vi "Get Cursor Info.vi"(8 "error in (no error)":errorcluster) -> (0 "error out":errorcluster, 1 "Image":T1, 2 "Hot Spot":cluster{"x":i32, "y":i32}, 3 "Position":cluster{"x":i32, "y":i32}, 4 "Drawn Image":picture)   [LabVIEW 2020, in "MacroAssert.lvlib" / "Win Util.lvlib"]
doc: "Originally found here.\n\nhttps://decibel.ni.com/content/docs/DOC-15261\n\nModified to get the image in a different way using the save to buffer, along with PNG conversion. Also got the position from the DLL call, and clear error if the data returned looks good.\n\n-----\nBrian Hoover (hooovahh)"
uses:
  Win Util.lvlib
  <vilib>/picture/picture.llb/imagedata.ctl
  System.Windows.Forms
  System.Drawing
  user32.dll
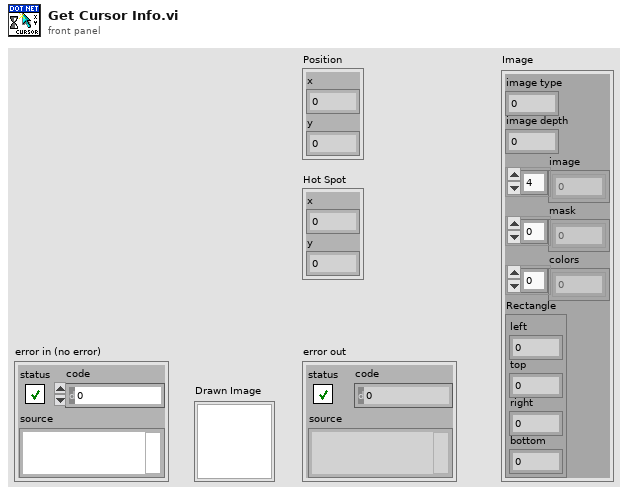
[diagram p1: front panel]
types:
  T1 = typedef "imagedata.ctl" = cluster{"image type":i32, "image depth":i32, "image":u8[], "mask":u8[], "colors":u32[], "Rectangle":cluster{"left":i16, "top":i16, "right":i16, "bottom":i16}}
  T2 = cluster{"cbSize":i32, "flags":i32, "HCURSOR":i32, "pos":cluster{"x":i32, "y":i32}}
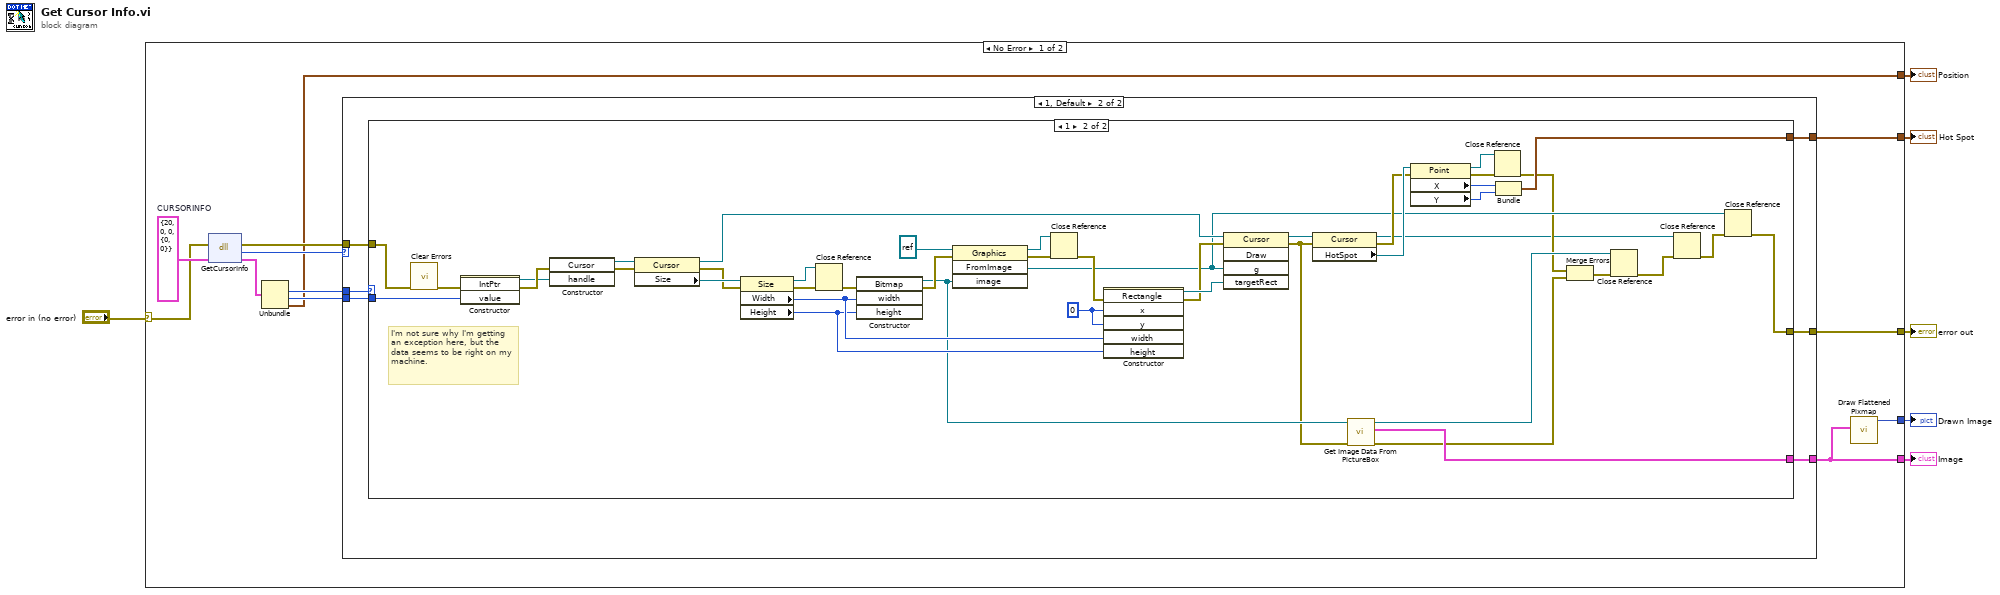
[diagram p0: block diagram]
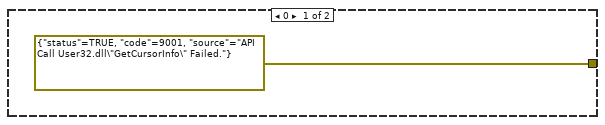
[diagram p2: hidden frame]
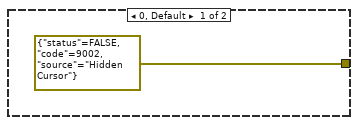
[diagram p3: hidden frame]
diagram:
  n1 = case shown="No Error" "error in (no error)" {
    selector: "error in (no error)" -> [w8 w70]
    tunnel: [w12 w70] -> w6
    tunnel: [w11 _] -> w5
    tunnel: [w10 _] -> w4
    tunnel: [w9 _] -> w3
    tunnel: [w7 _] -> w1
    frame No Error {
      w17 = T2 {"cbSize"=20, "flags"=0, "HCURSOR"=0, "pos"={"x"=0, "y"=0}}  # CURSORINFO
      n2 = dll-call lib="USER32.DLL" fn="GetCursorInfo"(error in=w8, w17) -> (error out=w13:errorcluster, "return type"=w15:i32, w18:T2)  [unwired: 2 in, 1 out]
      n3 = Unbundle(w18) -> ("flags"=w14:i32, "HCURSOR"=w16:i32, "pos"=w7:cluster{"x":i32, "y":i32})  [unwired: 1 out]
      n4 = case shown="1, Default" w15 {
        tunnel: w16 -> [_ w25]
        tunnel: [_ w24] -> w10
        tunnel: [errorcluster {"status"=TRUE, "code"=9001, "source"="API Call User32.dll\"GetCursorInfo\" Failed."} ("error out") w23] -> w12
        tunnel: [_ w22] -> w11
        tunnel: w14 -> [_ w21]
        tunnel: w13 -> [_ w20]
        frame 0 {
        }
        frame 1, Default {
          n5 = case shown="1" w21 {
            tunnel: w25 -> [_ w69]
            tunnel: [_ w68] -> w24
            tunnel: [errorcluster {"status"=FALSE, "code"=9002, "source"="Hidden Cursor"} ("error out") w60] -> w23
            tunnel: [_ w61] -> w22
            tunnel: w20 -> [_ w59]
            frame 0, Default {
            }
            frame 1 {
              w56 = 0 ("x")
              # "I'm not sure why I'm getting an exception here, but the data seems to be right on my machine."
              n6 = call <vilib>:"Clear Errors.vi"("error in (no error)"=w59) -> ("error out"=w57:errorcluster)  [unwired: 5 in, 1 out]
              n7 = constructor class="IntPtr"(error in=w57, "value"=w69) -> (reference out=w58:refnum<k24>, error out=w67:errorcluster)  [unwired: 2 in, 2 out]
              n8 = constructor class="Cursor"(error in=w67, "handle"=w58) -> (reference out=w65:refnum<k24>, error out=w66:errorcluster)  [unwired: 2 in, 2 out]
              n9 = property class="Cursor"(reference=w65, error in=w66) -> (reference out=w62:refnum<k24>, error out=w63:errorcluster, "Size"=w64:refnum<k24>)
              n10 = property class="Size"(reference=w64, error in=w63) -> (reference out=w54:refnum<k24>, error out=w55:errorcluster, "Width"=w52:i32, "Height"=w51:i32)
              n11 = Close Reference(reference=w54, error in (no error)=w55) -> (error out=w53:errorcluster)
              n12 = constructor class="Bitmap"(error in=w53, "width"=w52, "height"=w51) -> (reference out=w34:refnum<k24>, error out=w49:errorcluster)  [unwired: 2 in, 3 out]
              n13 = invoke class="Graphics" method="FromImage"(reference=refnum<k24> refnum ("new reference"), error in=w49, "image"=w34) -> (reference out=w45:refnum<k24>, error out=w46:errorcluster, "FromImage"=w36:refnum<k24>)  [unwired: 1 in, 1 out]
              n14 = Close Reference(reference=w45, error in (no error)=w46) -> (error out=w44:errorcluster)
              n15 = constructor class="Rectangle"(error in=w44, "x"=w56, "y"=w56, "width"=w52, "height"=w51) -> (reference out=w48:refnum<k24>, error out=w47:errorcluster)  [unwired: 2 in, 5 out]
              n16 = invoke class="Cursor" method="Draw"(reference=w62, error in=w47, "g"=w36, "targetRect"=w48) -> (reference out=w43:refnum<k24>, error out=w33:errorcluster)  [unwired: 1 in, 3 out]
              n17 = property class="Cursor"(reference=w43, error in=w33) -> (reference out=w27:refnum<k24>, error out=w41:errorcluster, "HotSpot"=w42:refnum<k24>)
              n18 = call "Get Image Data From PictureBox.vi"("error in (no error)"=w33, "Image"=w34) -> ("error out"=w31:errorcluster, "Image Data"=w68:T1, "Image Out"=w32:refnum<k24>)  [unwired: 7 in]
              n19 = property class="Point"(reference=w42, error in=w41) -> (reference out=w37:refnum<k24>, error out=w38:errorcluster, "X"=w40:i32, "Y"=w39:i32)
              n20 = Close Reference(reference=w37, error in (no error)=w38) -> (error out=w30:errorcluster)
              n21 = Bundle("X"=w40, "Y"=w39) -> (w61:cluster{"X":i32, "Y":i32})  [unwired: 1 in]
              n22 = Merge Errors(w30, w31) -> (w29:errorcluster)
              n23 = Close Reference(reference=w32, error in (no error)=w29) -> (error out=w28:errorcluster)
              n24 = Close Reference(reference=w27, error in (no error)=w28) -> (error out=w35:errorcluster)
              n25 = Close Reference(reference=w36, error in (no error)=w35) -> (error out=w60:errorcluster)
            }
          }
        }
      }
      n26 = call <vilib>:"Draw Flattened Pixmap.vi"("image data"=w10) -> ("new picture"=w9:picture)  [unwired: 8 in]
    }
    frame Error {
    }
  }
  "Image" <- w4
  "error out" <- w6
  "Hot Spot" <- w5
  "Drawn Image" <- w3
  "Position" <- w1
